vi "Configuration Dialog.vi"(3 "State in":T1={"Min Speed"=0.0, "Color"=0, "Max Speed"=100.0, "First Run?"=FALSE, "Value"=50.0, "Refnum"=refnum} caption="State") -> (0 "Cancelled?":bool, 1 "State out":T1 caption="State")   [LabVIEW 2012, in "Spinner.xctl"]
uses:
  Spinner.xctl
  Spinner State.ctl
  Command.ctl
panel:
  in  "error in":errorcluster
  out "error out":errorcluster
  in  "Value":dbl(slide)=50.0 scale=-60.0..60.0
  out "Spinner":picture
  in  "HELP":bool
  in  "Cancel":bool
  in  "OK":bool
  in  "Raw full speed":dbl=100.0 min=0.0
  in  "Raw zero speed":dbl min=0.0
  in  "Color":u32(colorbox)
  # "Preview"
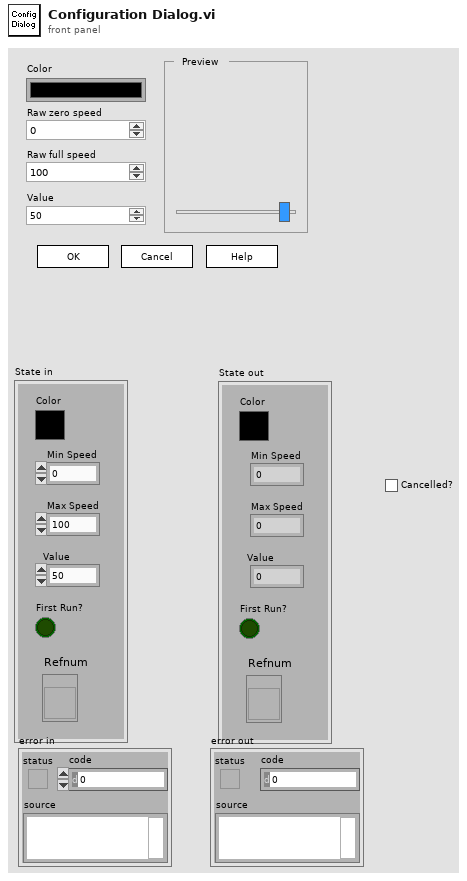
[diagram p1: front panel]
types:
  T1 = typedef "Spinner.xctl/Spinner State.ctl" = cluster{"Min Speed":dbl, "Color":u32, "Max Speed":dbl, "First Run?":bool, "Value":dbl, "Refnum":refnum<vi>}
  T2 = typedef "Spinner.xctl/Command.ctl" = enum16{"Add Control", "Remove Control", "Update Imgs", "Update Speed", "Refresh"}
  T3 = typedef "LVBoundsTypeDef.ctl" = cluster{"Width":u32, "Height":u32}
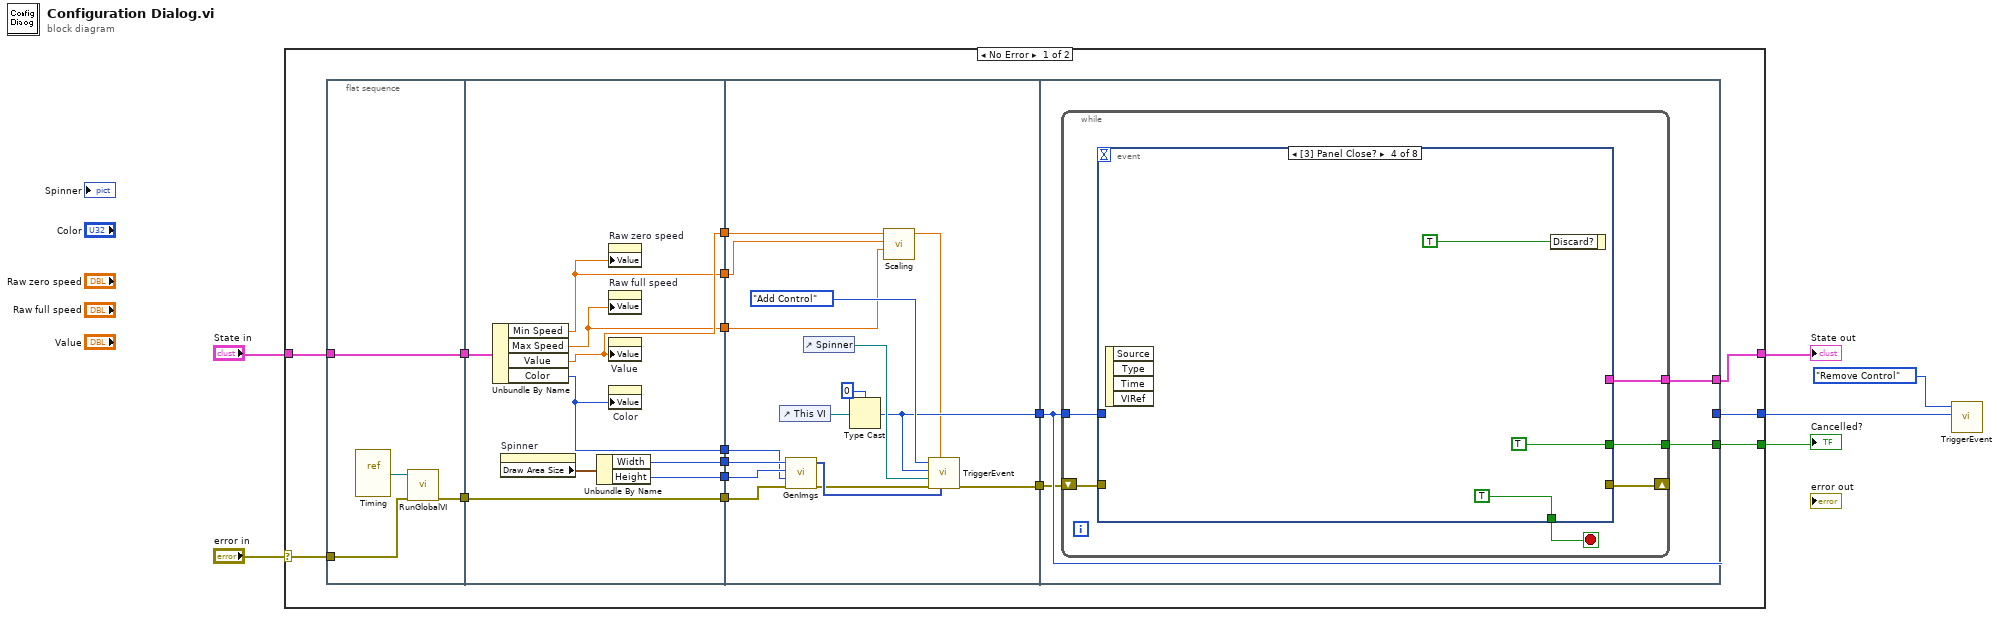
[diagram p0: block diagram]
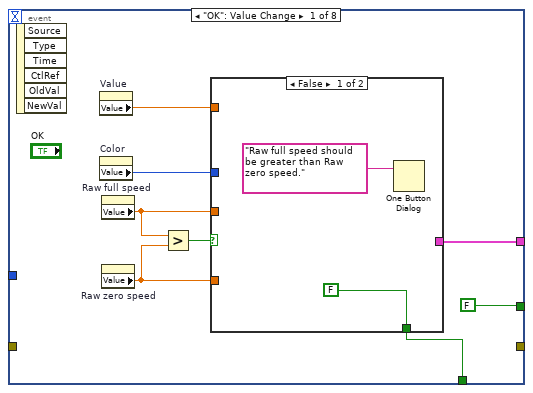
[diagram p2: hidden frame]
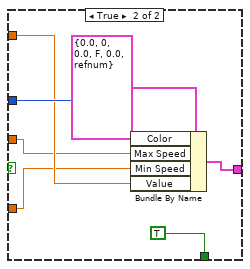
[diagram p3: hidden frame]
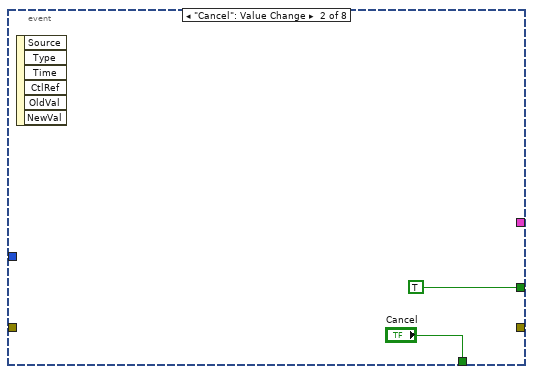
[diagram p4: hidden frame]
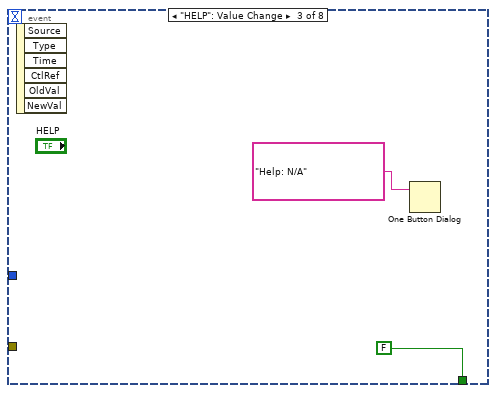
[diagram p5: hidden frame]
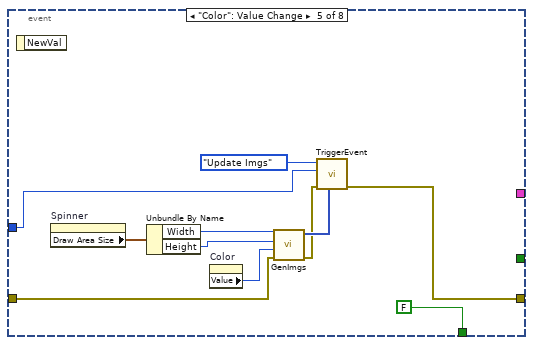
[diagram p6: hidden frame]
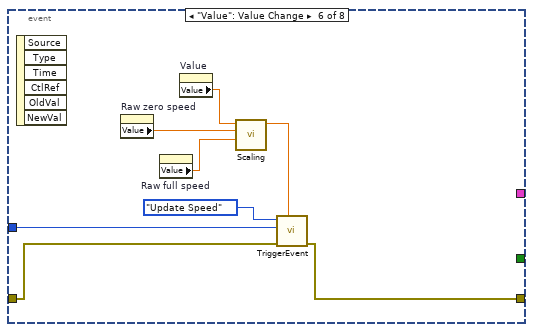
[diagram p7: hidden frame]
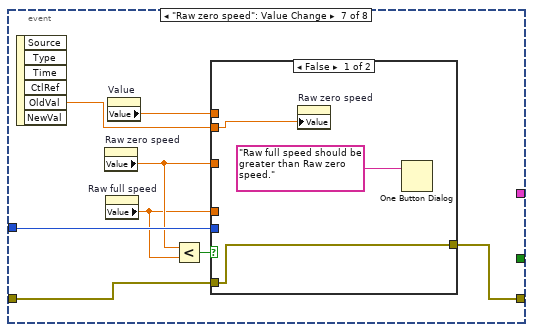
[diagram p8: hidden frame]
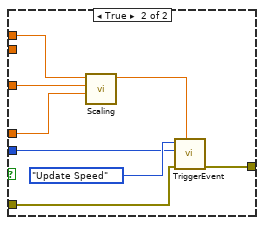
[diagram p9: hidden frame]
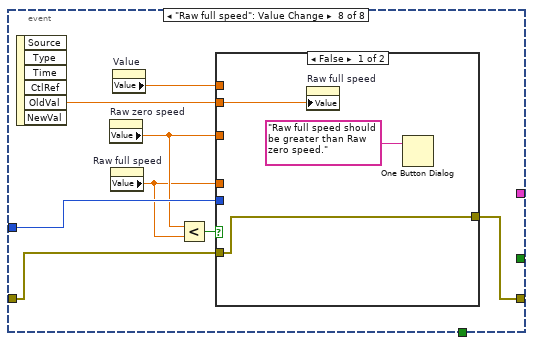
[diagram p10: hidden frame]
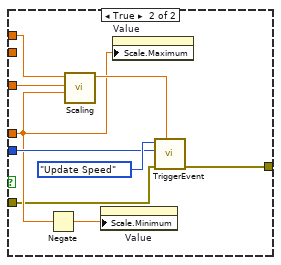
[diagram p11: hidden frame]
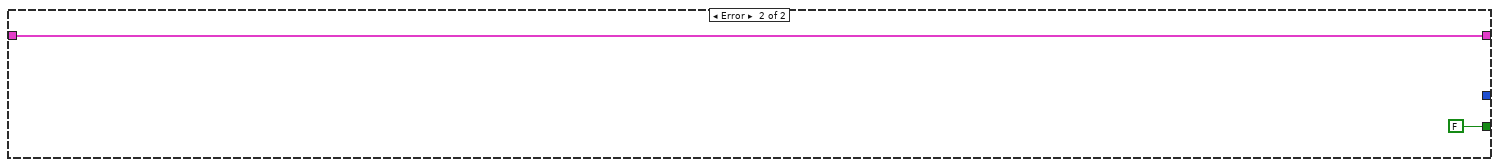
[diagram p12: hidden frame]
diagram:
  n1 = case shown="No Error" "error in" {
    selector: "error in" -> [w22 _]
    tunnel: "State in" -> [w20 w145]
    tunnel: [w13 _] -> w3
    tunnel: [w9 FALSE] -> w2
    tunnel: [w8 w145] -> w1
    frame No Error {
      n2 = flat-sequence {
        tunnel: w22 -> [w24]
        tunnel: [w25] -> w21
        tunnel: w20 -> [w25]
        tunnel: [w23] -> w15
        tunnel: w21 -> [w35]
        tunnel: [w33] -> w19
        tunnel: [w32] -> w18
        tunnel: [w31] -> w17
        tunnel: [w30] -> w16
        tunnel: w15 -> [w30]
        tunnel: [w29] -> w12
        tunnel: [w28] -> w11
        tunnel: [w27] -> w10
        tunnel: w19 -> [w47]
        tunnel: w18 -> [w46]
        tunnel: w17 -> [w45]
        tunnel: w16 -> [w44]
        tunnel: [w41] -> w14
        tunnel: w12 -> [w40]
        tunnel: w11 -> [w39]
        tunnel: w10 -> [w38]
        tunnel: [w36] -> w7
        tunnel: w14 -> [w55]
        tunnel: [w55] -> w13
        tunnel: [w54] -> w8
        tunnel: [w53] -> w9
        tunnel: w7 -> [w52]
        frame #0 {
          n3 = vi-ref "Timing.vi"() -> (w26:refnum<vi>)
          n4 = call "RunGlobalVI.vi"("error in"=w24, "VI input"=w26) -> ("error out"=w23:errorcluster)  [unwired: 9 in]
        }
        frame #1 {
          n5 = Unbundle By Name(w35) -> ("Min Speed"=w28:dbl, "Max Speed"=w27:dbl, "Value"=w29:dbl, "Color"=w31:u32)
          n6 = property on="Spinner" class="Pict"() -> ("Draw Area Size"=w34:T3)  [unwired: 2 in, 2 out]
          n7 = Unbundle By Name(w34) -> ("Width"=w33:u32, "Height"=w32:u32)
          n8 = property on="Raw zero speed" class="DigNum (strict)"("Value"=w28) -> ()  [unwired: 2 in, 2 out]
          n9 = property on="Raw full speed" class="DigNum (strict)"("Value"=w27) -> ()  [unwired: 2 in, 2 out]
          n10 = property on="Value" class="Slide (strict)"("Value"=w29) -> ()  [unwired: 2 in, 2 out]
          n11 = property on="Color" class="ColBox"("Value"=w31) -> ()  [unwired: 2 in, 2 out]
        }
        frame #2 {
          n12 = control-ref of="This VI"() -> (w51:refnum<vi>)
          n13 = call "GenImgs.vi"("error in"=w44, "Color"=w45, "Height"=w46, "Width"=w47) -> ("error out"=w42:errorcluster, "Imgs"=w43:picture[])  [unwired: 6 in]
          n14 = control-ref of="Spinner"() -> (w49:refnum<vi>)
          n15 = Type Cast(type=u32 0, x=w51) -> (*(type *) &x=w41:u32)
          n16 = call "Scaling.vi"("max"=w38, "min"=w39, "value"=w40) -> ("Length out"=w37:dbl)  [unwired: 7 in, 1 out]
          n17 = call "TriggerEvent.vi"("Imgs"=w43, "Step Len"=w37, "error in"=w42, "Pic Ref"=w49, "Ctrl Ref"=w41, "Command"=Command."Add Control") -> ("error out"=w36:errorcluster)  [unwired: 5 in]
        }
        frame #3 {
          n18 = while {
            tunnel: [w60] -> w53
            tunnel: [w59] -> w54
            tunnel: w55 -> [w58]
            shift-right: [w56] -> _
            shift-left: w52 -> [w57]
            stop <- w61 stop-if-true
            n19 = event shown="[3] Panel Close?" {
              selector: _ -> [_ _ _ _ _ _ _ _]
              dyn-events: _ -> [_ _ _ _ _ _ _ _]
              timeout: _ -> [_ _ _ _ _ _ _ _]
              tunnel: [w67 "Cancel" FALSE ("Cancel") TRUE FALSE ("Cancel") _ _ _] -> w61
              tunnel: [FALSE TRUE _ TRUE _ _ _ _] -> w60
              tunnel: [w68 _ _ _ _ _ _ _] -> w59
              tunnel: w58 -> [_ _ _ _ w92 w99 w111 w130]
              tunnel: w57 -> [_ _ _ _ w88 w98 w107 w126]
              tunnel: [_ _ _ _ w86 w97 w106 w125] -> w56
              event "OK": Value Change {
                n20 = event-data() -> ()  [unwired: 1 in, 6 out]
                n21 = property on="Value" class="Slide (strict)"() -> ("Value"=w62:dbl)  [unwired: 2 in, 2 out]
                n22 = property on="Color" class="ColBox"() -> ("Value"=w63:u32)  [unwired: 2 in, 2 out]
                n23 = property on="Raw full speed" class="DigNum (strict)"() -> ("Value"=w65:dbl)  [unwired: 2 in, 2 out]
                n24 = property on="Raw zero speed" class="DigNum (strict)"() -> ("Value"=w66:dbl)  [unwired: 2 in, 2 out]
                n25 = Greater?(x=w65, y=w66) -> (0:w64:bool)
                n26 = case shown="False" w64 {
                  tunnel: w66 -> [_ w73]
                  tunnel: w65 -> [_ w72]
                  tunnel: [_ w78] -> w68
                  tunnel: [FALSE TRUE] -> w67
                  tunnel: w63 -> [_ w75]
                  tunnel: w62 -> [_ w74]
                  frame False {
                    n27 = One Button Dialog(message="Raw full speed should be greater than Raw zero speed.") -> ()  [unwired: 1 in, 1 out]
                  }
                  frame True {
                    n28 = Bundle By Name(cluster=T1 {"Min Speed"=0.0, "Color"=0, "Max Speed"=0.0, "First Run?"=FALSE, "Value"=0.0, "Refnum"=refnum} ("State"), "Color"=w75, "Max Speed"=w72, "Min Speed"=w73, "Value"=w74) -> (w78:T1)
                  }
                }
              }
              event "Cancel": Value Change {
                n29 = event-data() -> ()  [unwired: 1 in, 6 out]
              }
              event "HELP": Value Change {
                n30 = event-data() -> ()  [unwired: 1 in, 6 out]
                n31 = One Button Dialog(message="Help: N/A") -> ()  [unwired: 1 in, 1 out]
              }
              event Panel Close? {
                n32 = event-data() -> ()  [unwired: 1 in, 4 out]
                n33 = event-data("Discard?"=TRUE) -> ()  [unwired: 1 in, 1 out]
              }
              event "Color": Value Change {
                n34 = event-data() -> ()  [unwired: 1 in, 1 out]
                n35 = property on="Spinner" class="Pict"() -> ("Draw Area Size"=w91:T3)  [unwired: 2 in, 2 out]
                n36 = Unbundle By Name(w91) -> ("Width"=w90:u32, "Height"=w89:u32)
                n37 = property on="Color" class="ColBox"() -> ("Value"=w94:u32)  [unwired: 2 in, 2 out]
                n38 = call "GenImgs.vi"("error in"=w88, "Color"=w94, "Height"=w89, "Width"=w90) -> ("error out"=w87:errorcluster, "Imgs"=w95:picture[])  [unwired: 6 in]
                n39 = call "TriggerEvent.vi"("Imgs"=w95, "error in"=w87, "Ctrl Ref"=w92, "Command"=Command."Update Imgs") -> ("error out"=w86:errorcluster)  [unwired: 7 in]
              }
              event "Value": Value Change {
                n40 = event-data() -> ()  [unwired: 1 in, 6 out]
                n41 = property on="Raw zero speed" class="DigNum (strict)"() -> ("Value"=w102:dbl)  [unwired: 2 in, 2 out]
                n42 = property on="Raw full speed" class="DigNum (strict)"() -> ("Value"=w101:dbl)  [unwired: 2 in, 2 out]
                n43 = property on="Value" class="Slide (strict)"() -> ("Value"=w103:dbl)  [unwired: 2 in, 2 out]
                n44 = call "Scaling.vi"("max"=w101, "min"=w102, "value"=w103) -> ("Length out"=w100:dbl)  [unwired: 7 in, 1 out]
                n45 = call "TriggerEvent.vi"("Step Len"=w100, "error in"=w98, "Ctrl Ref"=w99, "Command"=Command."Update Speed") -> ("error out"=w97:errorcluster)  [unwired: 7 in]
              }
              event "Raw zero speed": Value Change {
                n46 = event-data() -> ("OldVal"=w105:dbl)  [unwired: 1 in, 5 out]
                n47 = property on="Raw zero speed" class="DigNum (strict)"() -> ("Value"=w109:dbl)  [unwired: 2 in, 2 out]
                n48 = property on="Raw full speed" class="DigNum (strict)"() -> ("Value"=w108:dbl)  [unwired: 2 in, 2 out]
                n49 = property on="Value" class="Slide (strict)"() -> ("Value"=w112:dbl)  [unwired: 2 in, 2 out]
                n50 = Less?(x=w109, y=w108) -> (x < y?=w110:bool)
                n51 = case shown="False" w110 {
                  tunnel: w112 -> [_ w122]
                  tunnel: w109 -> [_ w118]
                  tunnel: w108 -> [_ w121]
                  tunnel: w111 -> [_ w119]
                  tunnel: w107 -> [w114 w117]
                  tunnel: [w114 w116] -> w106
                  tunnel: w105 -> [w113 _]
                  frame False {
                    n52 = property on="Raw zero speed" class="DigNum (strict)"("Value"=w113) -> ()  [unwired: 2 in, 2 out]
                    n53 = One Button Dialog(message="Raw full speed should be greater than Raw zero speed.") -> ()  [unwired: 1 in, 1 out]
                  }
                  frame True {
                    n54 = call "Scaling.vi"("max"=w121, "min"=w118, "value"=w122) -> ("Length out"=w120:dbl)  [unwired: 7 in, 1 out]
                    n55 = call "TriggerEvent.vi"("Step Len"=w120, "error in"=w117, "Ctrl Ref"=w119, "Command"=Command."Update Speed") -> ("error out"=w116:errorcluster)  [unwired: 7 in]
                  }
                }
              }
              event "Raw full speed": Value Change {
                n56 = event-data() -> ("OldVal"=w124:dbl)  [unwired: 1 in, 5 out]
                n57 = property on="Raw zero speed" class="DigNum (strict)"() -> ("Value"=w128:dbl)  [unwired: 2 in, 2 out]
                n58 = property on="Raw full speed" class="DigNum (strict)"() -> ("Value"=w127:dbl)  [unwired: 2 in, 2 out]
                n59 = property on="Value" class="Slide (strict)"() -> ("Value"=w131:dbl)  [unwired: 2 in, 2 out]
                n60 = Less?(x=w128, y=w127) -> (x < y?=w129:bool)
                n61 = case shown="False" w129 {
                  tunnel: w131 -> [_ w142]
                  tunnel: w128 -> [_ w139]
                  tunnel: w127 -> [_ w137]
                  tunnel: w130 -> [_ w140]
                  tunnel: w126 -> [w133 w136]
                  tunnel: [w133 w135] -> w125
                  tunnel: w124 -> [w132 _]
                  frame False {
                    n62 = property on="Raw full speed" class="DigNum (strict)"("Value"=w132) -> ()  [unwired: 2 in, 2 out]
                    n63 = One Button Dialog(message="Raw full speed should be greater than Raw zero speed.") -> ()  [unwired: 1 in, 1 out]
                  }
                  frame True {
                    n64 = Negate(x=w137) -> (-x=w138:dbl)
                    n65 = call "Scaling.vi"("max"=w137, "min"=w139, "value"=w142) -> ("Length out"=w141:dbl)  [unwired: 7 in, 1 out]
                    n66 = property on="Value" class="Slide (strict)"("Scale.Minimum"=w138) -> ()  [unwired: 2 in, 2 out]
                    n67 = property on="Value" class="Slide (strict)"("Scale.Maximum"=w137) -> ()  [unwired: 2 in, 2 out]
                    n68 = call "TriggerEvent.vi"("Step Len"=w141, "error in"=w136, "Ctrl Ref"=w140, "Command"=Command."Update Speed") -> ("error out"=w135:errorcluster)  [unwired: 7 in]
                  }
                }
              }
            }
          }
        }
      }
    }
    frame Error {
    }
  }
  "Cancelled?" <- w2
  "State out" <- w1
  n69 = call "TriggerEvent.vi"("Ctrl Ref"=w3, "Command"=Command."Remove Control") -> ()  [unwired: 9 in, 1 out]
